vi "Construct Temperature Forecast.vi"(5 "Temperature Forecast In":refnum<class "Temperature Forecast.lvclass">, 7 "Description":string, 8 "error in (no error)":errorcluster, 9 "Feels Like [°C]":dbl, 10 "Temperature [°C]":dbl, 11 "Date":timestamp) -> (0 "error out":errorcluster, 3 "Temperature Forecast":refnum<class "Temperature Forecast.lvclass">)   [LabVIEW 2017, in "Generic Object Serializer Tests.lvlib" / "Temperature Forecast.lvclass"]
uses:
  Temperature Forecast.lvclass
  C:/Users/de200256/Code/logmanoriginal/jsontext-object-serialization/Tests/Weather Forecast/Weather Forecast.lvclass
  Temperature Forecast.lvclass/Temperature Forecast.ctl
  Weather Forecast/Weather Forecast.lvclass
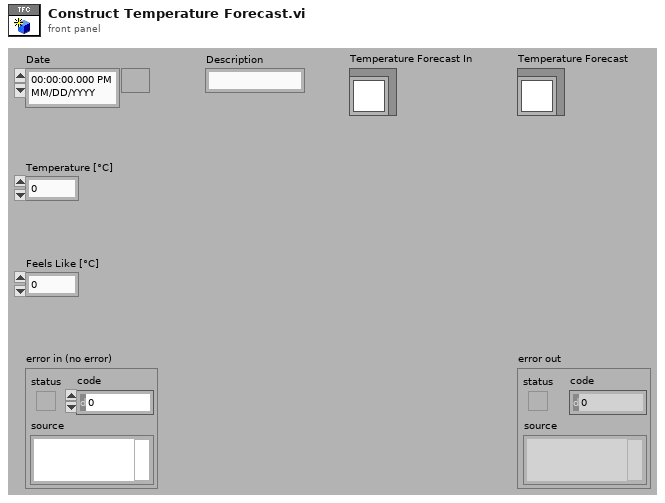
[diagram p1: front panel]
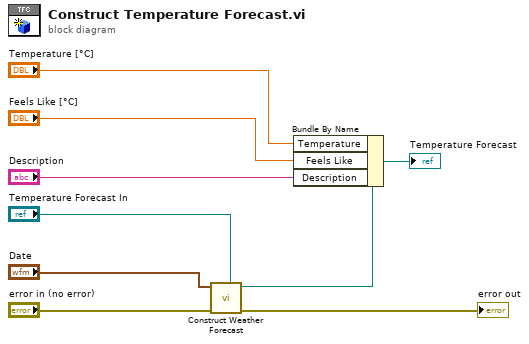
[diagram p0: block diagram]
diagram:
  n1 = call "Construct Weather Forecast.vi"("Weather Forecast In"="Temperature Forecast In", "error in (no error)"="error in (no error)", "Date"="Date") -> ("error out"=→"error out":errorcluster, "Weather Forecast"=w2:refnum<class "Temperature Forecast.lvclass">)  [unwired: 7 in]
  n2 = Bundle By Name(cluster=w2, "Temperature"="Temperature [°C]", "Feels Like"="Feels Like [°C]", "Description"="Description") -> (→"Temperature Forecast":refnum<class "Temperature Forecast.lvclass">)
